vi "Get Current Waveform.vi"(9 "Config":T1={"Channel Index"=1, "Shunt resistance"=0.001, "Channel name"="Heater Current"} {"Shunt resistance" format="%.4f"}, 11 "array":waveform(dbl)[](array[waveform])=[{"t0"=timestamp(3661870488.5173182 s since 1904-01-01), "dt"=0.001, "Y"=array[1000 elements], "attributes"=variant("NI_ChannelName"=variant(string "Heater Voltage"), "NI_UnitDescription"=variant(string "Volts"))}, {"t0"=timestamp(3661870488.517329 s since 1904-01-01), "dt"=0.001, "Y"=array[1000 elements], "attributes"=variant("NI_ChannelName"=variant(string "Heater Shunt"), "NI_UnitDescription"=variant(string "Volts"))}, {"t0"=timestamp(3661870488.51734 s since 1904-01-01), "dt"=0.001, "Y"=array[1000 elements], "attributes"=variant("NI_ChannelName"=variant(string "Diode Voltage"), "NI_UnitDescription"=variant(string "Volts"))}, {"t0"=timestamp(3661870488.517351 s since 1904-01-01), "dt"=0.001, "Y"=array[1000 elements], "attributes"=variant("NI_ChannelName"=variant(string "Thermopile Voltage"), "NI_UnitDescription"=variant(string "Volts"))}]) -> (1 "Channel name":string="Heater Shunt", 3 "Current waveform out":waveform(dbl)={"t0"=timestamp(3661870488.517329 s since 1904-01-01), "dt"=0.001, "Y"=array[1000 elements], "attributes"=variant("NI_ChannelName"=variant(string "Heater Current"), "NI_UnitDescription"=variant(string "A"))})   [LabVIEW 2019]
doc: "This example demonstrates how to acquire a continuous amount of data (Waveform) using the DAQ device's internal clock. It also shows how to synchronize two devices for different device families (E Series, S Series, M Series, X Series, DSA, and SC Express), to simultaneously acquire the data.\n\nFor instructions on how to connect your signals to the DAQ device, refer to your device documentation."
panel:
  # "Get Current Waveform"
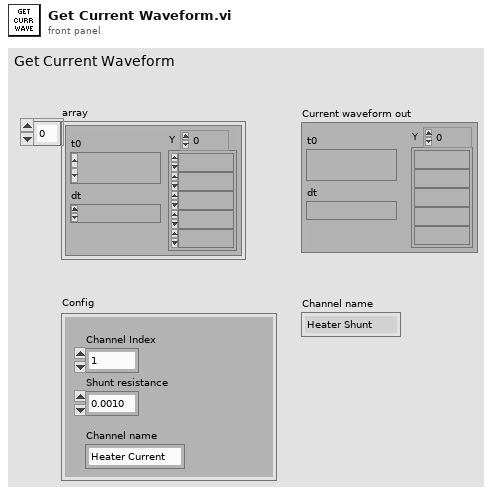
[diagram p1: front panel]
types:
  T1 = cluster{"Channel Index":i32, "Shunt resistance":dbl, "Channel name":string}
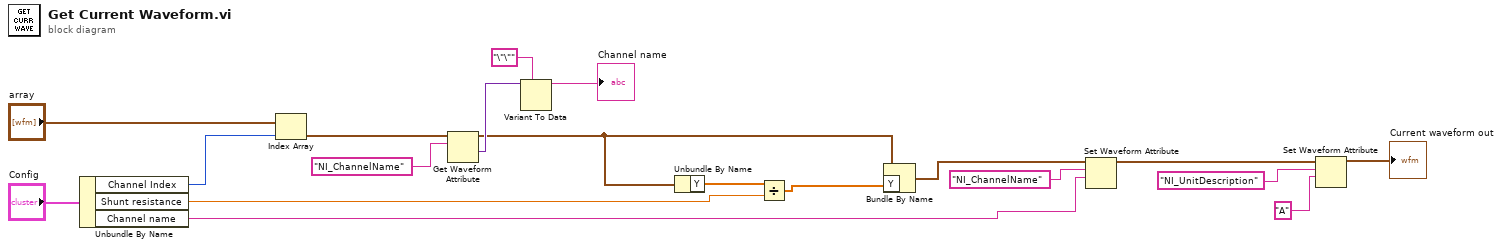
[diagram p0: block diagram]
diagram:
  n1 = Unbundle By Name("Config") -> ("Channel Index"=w10:i32, "Shunt resistance"=w3:dbl, "Channel name"=w5:string)
  n2 = Index Array(array="array", index=w10) -> (element=w14:waveform(dbl))
  n3 = Get Waveform Attribute(6:"NI_ChannelName" ("name"), 7:w14) -> (1:w8:variant, 3:w6:waveform(dbl))  [unwired: 2 in, 2 out]
  n4 = Variant To Data(type="\"\"" ("name"), Variant=w8) -> (data=→"Channel name":string)  [unwired: 1 in, 1 out]
  n5 = Unbundle By Name(w6) -> ("Y"=w4:dbl[])
  n6 = Divide(x=w4, y=w3) -> (x/y=w1:dbl[])
  n7 = Bundle By Name(cluster=w6, "Y"=w1) -> (w2:waveform(dbl))
  n8 = Set Waveform Attribute(5:w5, 6:"NI_ChannelName" ("name"), 7:w2) -> (3:w16:waveform(dbl))  [unwired: 1 in, 2 out]
  n9 = Set Waveform Attribute(5:"A" ("name"), 6:"NI_UnitDescription" ("name"), 7:w16) -> (3:→"Current waveform out":waveform(dbl))  [unwired: 1 in, 2 out]
